vi "FitAndSubtract.vi"(6 "Array 4":i16[](array[numeric]), 9 "Array 3":dbl[](array[numeric]), 10 "Numeric":i32, 11 "Array in":dbl[](array[numeric])) -> (2 "Best Polynomial Fit":dbl[](array[numeric]), 3 "Array out":dbl[](array[numeric]))   [LabVIEW 2019]
uses:
  <vilib>/Analysis/NI_AALPro.lvlib
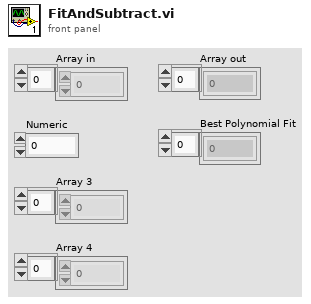
[diagram p1: front panel]
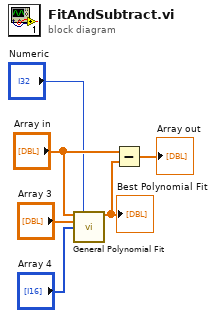
[diagram p0: block diagram]
diagram:
  n1 = call <vilib>:"General Polynomial Fit.vi"("Y"="Array in", "polynomial order"="Numeric", "X"="Array 3", "Weight"="Array 4") -> ("Best Polynomial Fit"=w5:dbl[])  [unwired: 8 in, 3 out]
  "Best Polynomial Fit" <- w5
  n2 = Subtract(x="Array in", y=w5) -> (x-y=→"Array out":dbl[])
